vi "MPS_Bed_control.vi"(8 "Motor speed":string(combo)="Sixteenth step", 9 "pulse duration (T/2)":dbl=0.0015 format="%#_13p", 10 "Sequence to run on start up":string[](array[string]), 11 "Signed pulses to move":dbl=1000.0) -> ()   [LabVIEW 2021]
uses:
  <vilib>/DAQmx/write.llb/DAQmx Write (Digital 1D Wfm NChan NSamp).vi
  <vilib>/DAQmx/read.llb/DAQmx Read (Digital Bool 1Line 1Point).vi
  <vilib>/Waveform/DWDTOps.llb/DWDT Digital Size.vi
  <vilib>/DAQmx/create/channels.llb/DAQmx Create Channel (DO-Digital Output).vi
  <vilib>/DAQmx/configure/timing.llb/DAQmx Timing (Sample Clock).vi
  <vilib>/Waveform/DWDTOps.llb/DWDT Uncompress Digital.vi
  <vilib>/DAQmx/miscellaneous.llb/DAQmx Fill In Error Info.vi
  <vilib>/DAQmx/create/channels.llb/DAQmx Create Channel (DI-Digital Input).vi
panel:
  out "Pulses traveled":dbl
  out "Duration of equivalent pulse":dbl
  out "Speed Mode":i32=16
  out "Steps to home":i32
  out "Homing switch":bool=TRUE
  in  "Homing Line":tag="H1/port0/line5"
  in  "lines":tag="H1/port0/line0:4"
  out "Main loop has stopped":bool
  out "Last system state called":string="Post homing"
  in  "pulse steps":dbl=10.0 min=0.0 step=1.0 format="%#_6p"
  in  "Move bed 2":bool
  out "Homing in progress":bool
  out "duration of movement":dbl=256.0
  in  "Maximum absolute position":i32=250 format="%.0p"
  in  "Abort movement":bool
  in  "Go home!":bool
  in  "Move bed":bool
  in  "Halt":bool
  # "For programatical use only!\nEnsure that the sequence control is empty before setting default values!"
  # "Homing"
  # "Enables PDU automatically"
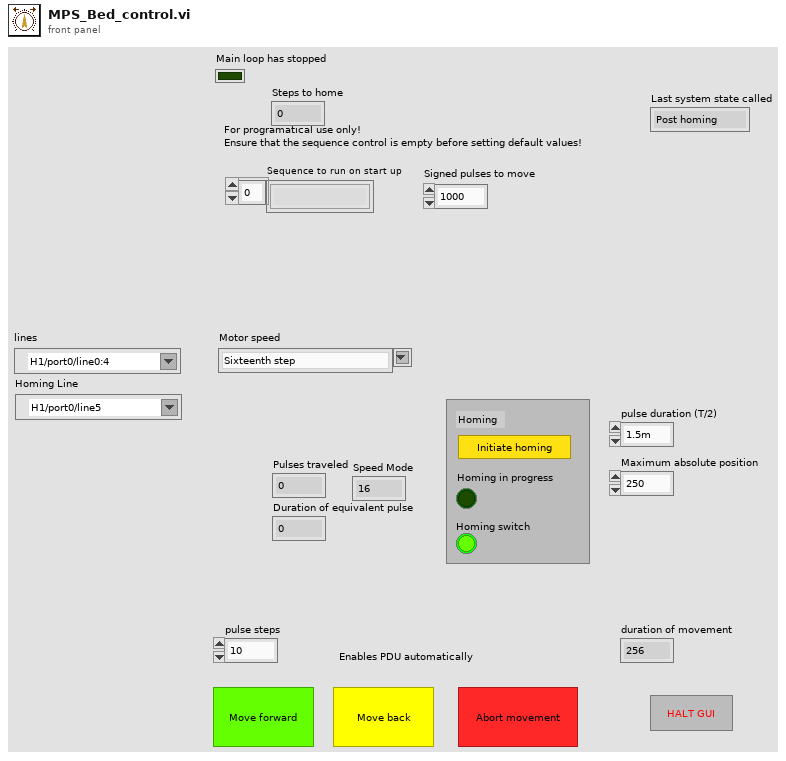
[diagram p1: front panel]
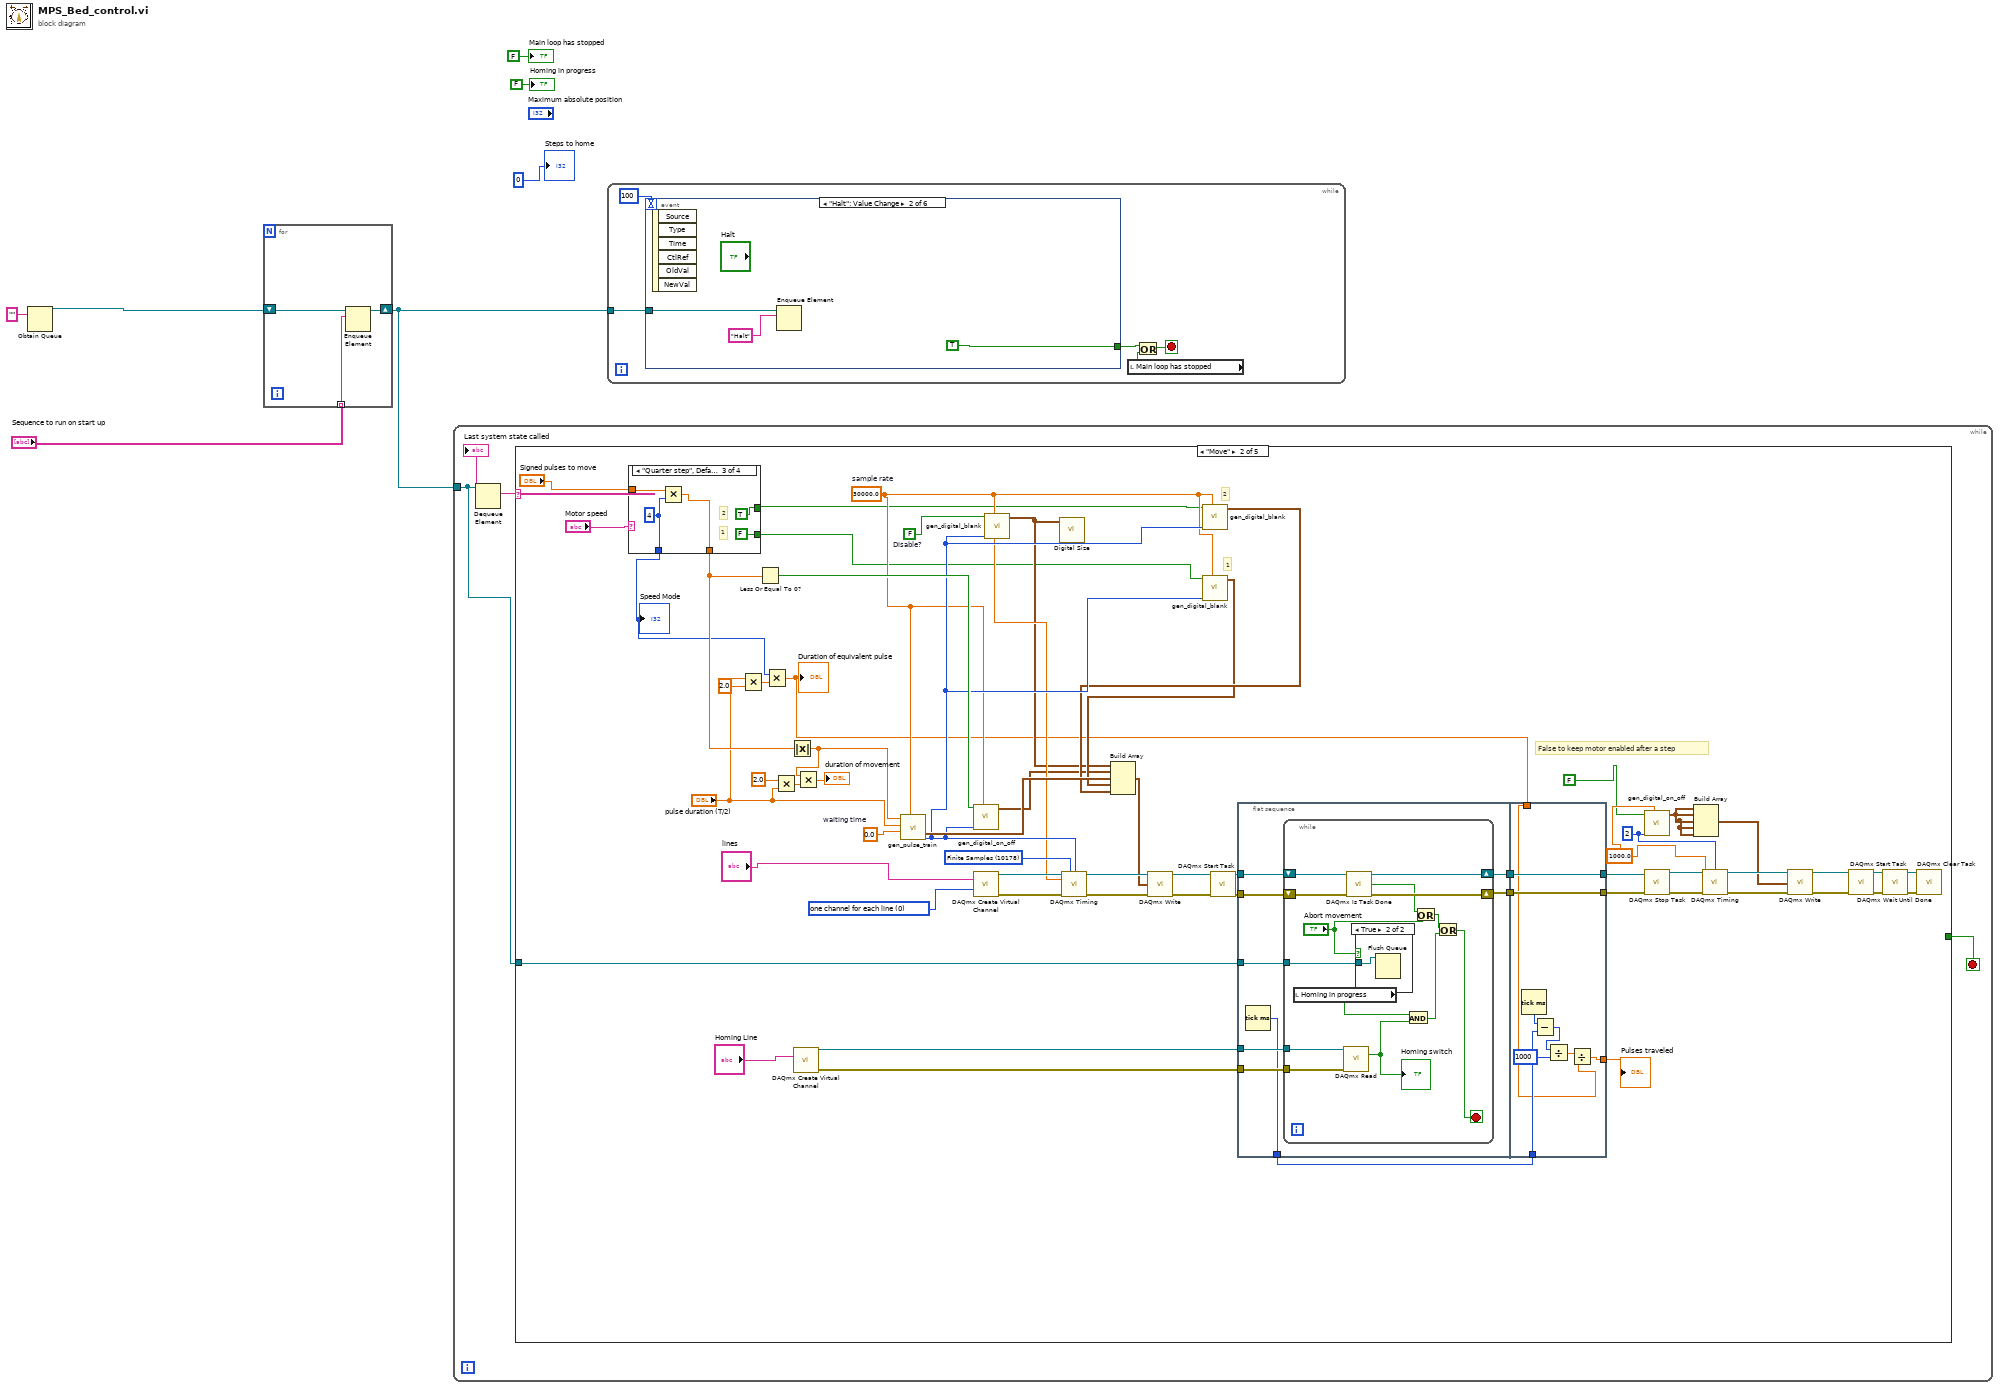
[diagram p0: block diagram]
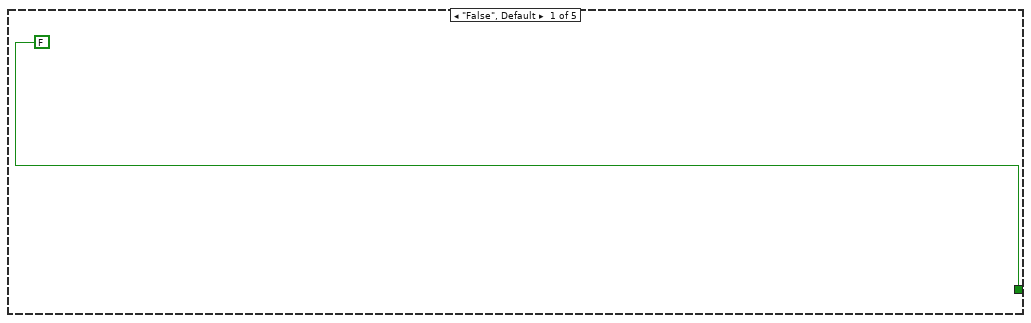
[diagram p2: hidden frame]
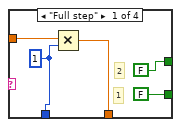
[diagram p4: hidden frame]
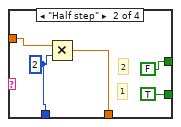
[diagram p5: hidden frame]
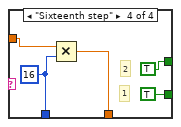
[diagram p6: hidden frame]
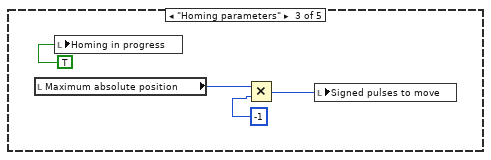
[diagram p7: hidden frame]
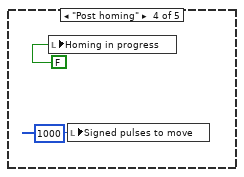
[diagram p8: hidden frame]
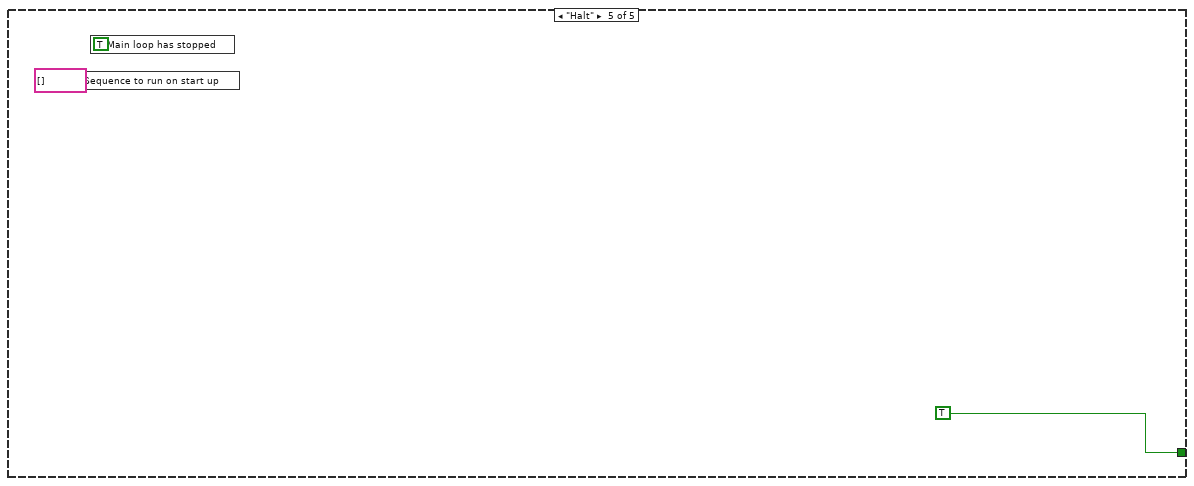
[diagram p9: hidden frame]
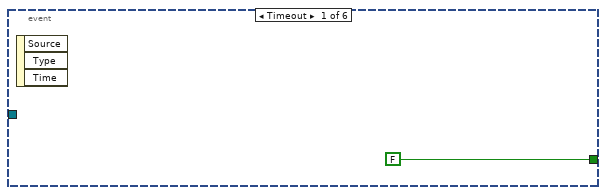
[diagram p10: hidden frame]
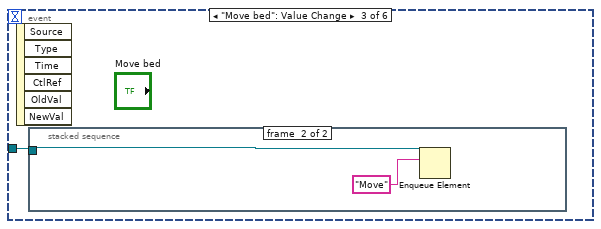
[diagram p11: hidden frame]
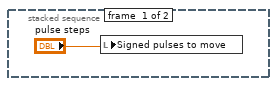
[diagram p12: hidden frame]
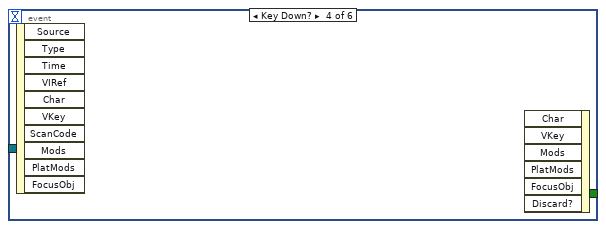
[diagram p13: hidden frame]
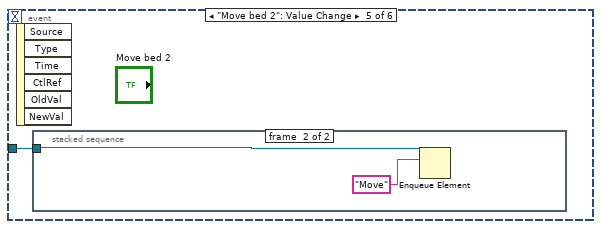
[diagram p14: hidden frame]
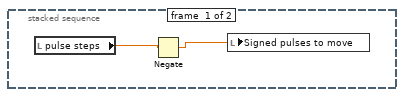
[diagram p15: hidden frame]
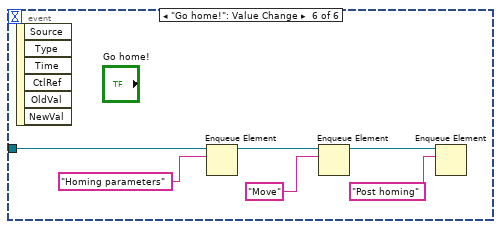
[diagram p16: hidden frame]
diagram:
  n1 = Obtain Queue(element data type="") -> (queue out=w2:refnum<queue>)  [unwired: 4 in, 2 out]
  n2 = for {
    shift-right: [w9] -> w5
    shift-left: w2 -> [w10]
    tunnel: "Sequence to run on start up" -> [w8] mode=indexing
    n3 = Enqueue Element(queue=w10, element=w8) -> (queue out=w9:refnum<queue>)  [unwired: 2 in, 2 out]
  }
  n4 = while {
    tunnel: w5 -> [w11]
    stop <- w12 stop-if-true
    n5 = Dequeue Element(queue=w11) -> (element=w13:string)  [unwired: 2 in, 3 out]
    "Last system state called" <- w13
    n6 = case shown="\"Move\"" w13 {
      tunnel: [FALSE _ _ _ TRUE] -> w12
      tunnel: w11 -> [_ w28 _ _ _]
      frame "False", Default {
      }
      frame "Move" {
        w43 = 2 ("waveform length")
        w44 = 1000.0 ("rate")
        w65 = 0.0  # waiting time
        w38 = 30000.0  # sample rate
        w68 = FALSE  # Disable?
        w67 = 10178 items=["Finite Samples"=10178, "Continuous Samples"=10123, "Hardware Timed Single Point"=12522] ("sample mode")
        w66 = 0 items=["one channel for each line", "one channel for all lines"] ("line grouping")
        # "1"
        # "2"
        # "False to keep motor enabled after a step"
        n7 = case shown="\"Quarter step\", Default" "Motor speed" {
          tunnel: "Signed pulses to move" -> [w112 w117 w122 w127]
          tunnel: [FALSE ("motor speed control 1") FALSE ("motor speed control 1") TRUE ("motor speed control 1") TRUE ("motor speed control 1")] -> w32
          tunnel: [FALSE ("motor speed control 1") TRUE ("motor speed control 1") FALSE ("motor speed control 1") TRUE ("motor speed control 1")] -> w31
          tunnel: [w109 w114 w119 w124] -> w30
          tunnel: [w108 w113 w118 w123] -> w17
          frame "Full step" {
            w108 = 1 ("y")
            # "1"
            # "2"
            n8 = Multiply(x=w112, y=w108) -> (x*y=w109:dbl)
          }
          frame "Half step" {
            w113 = 2 ("y")
            # "1"
            # "2"
            n9 = Multiply(x=w117, y=w113) -> (x*y=w114:dbl)
          }
          frame "Quarter step", Default {
            w118 = 4 ("y")
            # "1"
            # "2"
            n10 = Multiply(x=w122, y=w118) -> (x*y=w119:dbl)
          }
          frame "Sixteenth step" {
            w123 = 16 ("y")
            # "1"
            # "2"
            n11 = Multiply(x=w127, y=w123) -> (x*y=w124:dbl)
          }
        }
        "Speed Mode" <- w17
        n12 = Multiply(x="pulse duration (T/2)", y=2.0) -> (x*y=w18:dbl)
        n13 = Less Or Equal To 0?(x=w30) -> (x <= 0?=w64:bool)
        n14 = Multiply(x=w17, y=w18) -> (x*y=w16:dbl)
        "Duration of equivalent pulse" <- w16
        n15 = Multiply(x=2.0, y="pulse duration (T/2)") -> (x*y=w61:dbl)
        n16 = Absolute Value(x=w30) -> (abs(x)=w62:dbl)
        n17 = call-poly <vilib>:"DAQmx Create Virtual Channel.vi"("lines"="Homing Line") -> ("task out"=w26:refnum<k21>, "error out"=w25:errorcluster)  [unwired: 13 in]
        n18 = Multiply(x=w62, y=w61) -> (x*y=→"duration of movement":dbl)
        n19 = call "gen_pulse_train.vi"("sampling rate"=w38, "waiting time"=w65, "pulse width"="pulse duration (T/2)", "Number of pulses"=w62) -> ("waveform length"=w40:i32, "digital waveform out"=w73:digitalwaveform)  [unwired: 6 in]
        n20 = call "gen_digital_on_off.vi"("sampling rate"=w38, "waveform length"=w40, "On / Off"=w64) -> ("digital waveform"=w34:digitalwaveform)  [unwired: 8 in]
        n21 = call-poly <vilib>:"DAQmx Create Virtual Channel.vi"("lines"="lines", "line grouping"=w66) -> ("task out"=w69:refnum<k21>, "error out"=w72:errorcluster)  [unwired: 12 in]
        n22 = call "gen_digital_blank.vi"("sampling rate"=w38, "waveform length"=w40, "On / Off"=w68) -> ("digital waveform"=w35:digitalwaveform)  [unwired: 8 in]
        n23 = call-poly <vilib>:"Digital Size.vi"("digital waveform in"=w35) -> ()  [unwired: 7 in, 4 out]
        n24 = call-poly <vilib>:"DAQmx Timing.vi"("task/channels in"=w69, "sample mode"=w67, "samples per channel"=w40, "rate"=w38, "error in"=w72) -> ("task out"=w70:refnum<k21>, "error out"=w71:errorcluster)  [unwired: 9 in]
        n25 = call "gen_digital_blank.vi"("sampling rate"=w38, "waveform length"=w40, "On / Off"=w32) -> ("digital waveform"=w37:digitalwaveform)  [unwired: 8 in]
        n26 = call "gen_digital_blank.vi"("sampling rate"=w38, "waveform length"=w40, "On / Off"=w31) -> ("digital waveform"=w36:digitalwaveform)  [unwired: 8 in]
        n27 = Build Array(w35, w34, w73, w36, w37) -> (w42:digitalwaveform[])
        n28 = call-poly <vilib>:"DAQmx Write.vi"("task/channels in"=w70, "data"=w42, "error in"=w71) -> ("task out"=w74:refnum<k21>, "error out"=w75:errorcluster)  [unwired: 10 in, 1 out]
        n29 = call <vilib>:"DAQmx Start Task.vi"("task/channels in"=w74, "error in"=w75) -> ("task out"=w59:refnum<k21>, "error out"=w58:errorcluster)  [unwired: 12 in]
        n30 = flat-sequence {
          tunnel: w59 -> [w83]
          tunnel: w58 -> [w82]
          tunnel: w28 -> [w79]
          tunnel: w26 -> [w78]
          tunnel: w25 -> [w77]
          tunnel: [w81] -> w23
          tunnel: [w80] -> w22
          tunnel: [w76] -> w21
          tunnel: [w106] -> w56
          tunnel: [w107] -> w57
          tunnel: w23 -> [w107]
          tunnel: w22 -> [w106]
          tunnel: w21 -> [w105]
          tunnel: w16 -> [w100]
          tunnel: [w99] -> w15
          frame #0 {
            n31 = Tick Count (ms)() -> (millisecond timer value=w76:u32)
            n32 = while {
              shift-right: [w94] -> w80
              shift-left: w82 -> [w96]
              shift-right: [w95] -> w81
              shift-left: w83 -> [w97]
              tunnel: w79 -> [w87]
              tunnel: w78 -> [w85]
              tunnel: w77 -> [w84]
              stop <- w91 stop-if-true
              n33 = local read "Homing in progress"() -> (w90:bool)
              n34 = call-poly <vilib>:"DAQmx Read.vi"("task/channels in"=w85, "error in"=w84) -> ("data"=w86:bool)  [unwired: 11 in, 2 out]
              "Homing switch" <- w86
              n35 = call <vilib>:"DAQmx Is Task Done.vi"("task/channels in"=w97, "error in"=w96) -> ("task out"=w95:refnum<k21>, "task done?"=w93:bool, "error out"=w94:errorcluster)  [unwired: 11 in]
              n36 = case shown="True" "Abort movement" {
                tunnel: w87 -> [_ w98]
                frame False {
                }
                frame True {
                  n37 = Flush Queue(queue=w98) -> ()  [unwired: 1 in, 3 out]
                }
              }
              n38 = And(x=w90, y=w86) -> (x .and. y?=w89:bool)
              n39 = Or(x=w93, y="Abort movement") -> (x .or. y?=w92:bool)
              n40 = Or(x=w92, y=w89) -> (x .or. y?=w91:bool)
            }
          }
          frame #1 {
            n41 = Tick Count (ms)() -> (millisecond timer value=w104:u32)
            n42 = Subtract(x=w104, y=w105) -> (x-y=w103:u32)
            n43 = Divide(x=w103, y=u32 1000) -> (x/y=w101:dbl)
            n44 = Divide(x=w101, y=w100) -> (x/y=w99:dbl)
          }
        }
        n45 = call "gen_digital_on_off.vi"("sampling rate"=w44, "waveform length"=w43, "On / Off"=FALSE ("Keep enabled\n(inverted logic)")) -> ("digital waveform"=w39:digitalwaveform)  [unwired: 8 in]
        n46 = call <vilib>:"DAQmx Stop Task.vi"("task/channels in"=w57, "error in"=w56) -> ("task out"=w46:refnum<k21>, "error out"=w49:errorcluster)  [unwired: 12 in]
        n47 = Build Array(w39, w39, w39, w39, w39) -> (w45:digitalwaveform[])
        n48 = call-poly <vilib>:"DAQmx Timing.vi"("task/channels in"=w46, "samples per channel"=w43, "rate"=w44, "error in"=w49) -> ("task out"=w47:refnum<k21>, "error out"=w48:errorcluster)  [unwired: 10 in]
        n49 = call-poly <vilib>:"DAQmx Write.vi"("task/channels in"=w47, "data"=w45, "error in"=w48) -> ("task out"=w55:refnum<k21>, "error out"=w54:errorcluster)  [unwired: 10 in, 1 out]
        n50 = call <vilib>:"DAQmx Start Task.vi"("task/channels in"=w55, "error in"=w54) -> ("task out"=w53:refnum<k21>, "error out"=w52:errorcluster)  [unwired: 12 in]
        n51 = call <vilib>:"DAQmx Wait Until Done.vi"("task/channels in"=w53, "error in"=w52) -> ("task out"=w51:refnum<k21>, "error out"=w50:errorcluster)  [unwired: 12 in]
        n52 = call <vilib>:"DAQmx Clear Task.vi"("task in"=w51, "error in"=w50) -> ()  [unwired: 13 in, 1 out]
        "Pulses traveled" <- w15
      }
      frame "Homing parameters" {
        n53 = local read "Maximum absolute position"() -> (w130:i32)
        n54 = local write "Homing in progress"(TRUE ("Homing in progress")) -> ()
        n55 = Multiply(x=w130, y=-1) -> (x*y=w128:i32)
        n56 = local write "Signed pulses to move"(w128) -> ()
      }
      frame "Post homing" {
        n57 = local write "Homing in progress"(FALSE ("Homing in progress")) -> ()
        n58 = local write "Signed pulses to move"(1000 ("pulses to move")) -> ()
      }
      frame "Halt" {
        n59 = local write "Sequence to run on start up"(string[] [] ("Sequence to run on start up")) -> ()
        n60 = local write "Main loop has stopped"(TRUE ("Main loop has stopped")) -> ()
      }
    }
  }
  n61 = while {
    tunnel: w5 -> [w141]
    stop <- w138 stop-if-true
    n62 = event shown="[1] \"Halt\": Value Change" {
      selector: _ -> [_ _ _ _ _ _]
      dyn-events: _ -> [_ _ _ _ _ _]
      timeout: 100 -> [_ _ _ _ _ _]
      tunnel: w141 -> [_ w145 w146 _ w150 w159]
      tunnel: [FALSE TRUE _ _ _ _] -> w139
      event Timeout {
        n63 = event-data() -> ()  [unwired: 1 in, 3 out]
      }
      event "Halt": Value Change {
        n64 = event-data() -> ()  [unwired: 1 in, 6 out]
        n65 = Enqueue Element(queue=w145, element="Halt") -> ()  [unwired: 2 in, 3 out]
      }
      event "Move bed": Value Change {
        n66 = event-data() -> ()  [unwired: 1 in, 6 out]
        n67 = stacked-sequence {
          tunnel: w146 -> [_ w148]
          frame #0 {
            n68 = local write "Signed pulses to move"("pulse steps") -> ()
          }
          frame #1 {
            n69 = Enqueue Element(queue=w148, element="Move") -> ()  [unwired: 2 in, 3 out]
          }
        }
      }
      event Key Down? {
        n70 = event-data() -> ()  [unwired: 1 in, 10 out]
        n71 = event-data() -> ()  [unwired: 7 in, 1 out]
      }
      event "Move bed 2": Value Change {
        n72 = event-data() -> ()  [unwired: 1 in, 6 out]
        n73 = stacked-sequence {
          tunnel: w150 -> [_ w153]
          frame #0 {
            n74 = local read "pulse steps"() -> (w151:dbl)
            n75 = Negate(x=w151) -> (-x=w152:dbl)
            n76 = local write "Signed pulses to move"(w152) -> ()
          }
          frame #1 {
            n77 = Enqueue Element(queue=w153, element="Move") -> ()  [unwired: 2 in, 3 out]
          }
        }
      }
      event "Go home!": Value Change {
        n78 = event-data() -> ()  [unwired: 1 in, 6 out]
        n79 = Enqueue Element(queue=w159, element="Homing parameters") -> (queue out=w157:refnum<queue>)  [unwired: 2 in, 2 out]
        n80 = Enqueue Element(queue=w157, element="Move") -> (queue out=w155:refnum<queue>)  [unwired: 2 in, 2 out]
        n81 = Enqueue Element(queue=w155, element="Post homing") -> ()  [unwired: 2 in, 3 out]
      }
    }
    n82 = local read "Main loop has stopped"() -> (w140:bool)
    n83 = Or(x=w139, y=w140) -> (x .or. y?=w138:bool)
  }
  "Homing in progress" <- FALSE ("Homing in progress")
  "Main loop has stopped" <- FALSE ("Main loop has stopped")
  "Steps to home" <- 0
